vi "CameraGetData.vi"(7 "Action":T1, 8 "error in":errorcluster, 10 "element data type":variant, 11 "name (unnamed)":string) -> (0 "error out":errorcluster, 2 "notifier out":refnum<notifier>)   [LabVIEW 2013]
doc: "NotifierWrapper stores a notifier and allows the user to perform actions on it.\n-Init: create a new notifier with the given data type and name.\n-Get: return a reference to the notifier."
uses:
  QueueAction.ctl
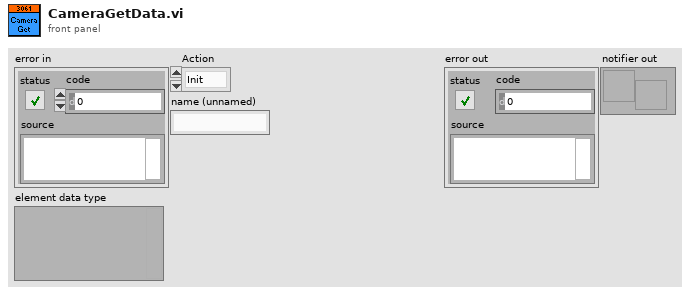
[diagram p1: front panel]
types:
  T1 = typedef "QueueAction.ctl" = enum16{"Init", "Get"}
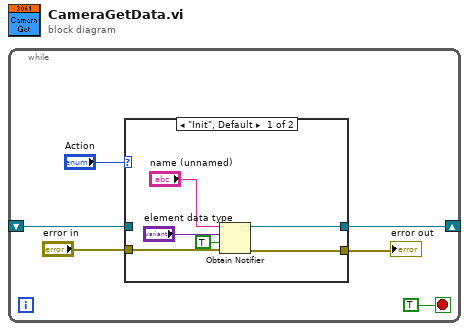
[diagram p0: block diagram]
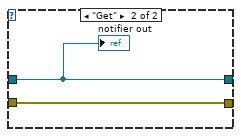
[diagram p2: hidden frame]
diagram:
  n1 = while {
    shift-right: [w2] -> _
    shift-left: _ -> [w1]
    stop <- TRUE stop-if-true
    n2 = case shown="\"Init\", Default" "Action" {
      tunnel: "error in" -> [w12 w13]
      tunnel: [w9 w13] -> w3
      tunnel: [w8 w14] -> w2
      tunnel: w1 -> [_ w14]
      frame "Init", Default {
        n3 = Obtain Notifier(name (unnamed)="name (unnamed)", notification data type="element data type", create if not found? (T)=TRUE, error in (no error)=w12) -> (notifier out=w8:refnum<notifier>, error out=w9:errorcluster)  [unwired: 1 out]
      }
      frame "Get" {
        "notifier out" <- w14
      }
    }
    "error out" <- w3
  }
